vi "Set String Constant Value.vi"(8 "Error In":errorcluster, 9 "Value":string, 10 "Label":string, 11 "VI Path":path) -> (0 "Error Out":errorcluster)   [LabVIEW 2011, in "Generator.lvlib"]
doc: "This VI sets the value of a labeled string constant."
uses:
  Generator.lvlib
  <vilib>/Utility/traverseref.llb/TRef TravTarget.ctl
  <vilib>/Utility/traverseref.llb/VI Scripting - Traverse.lvlib
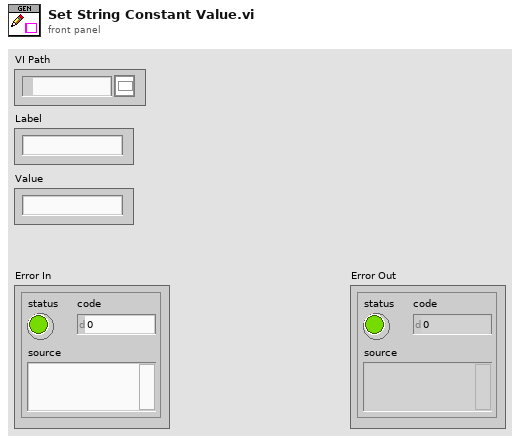
[diagram p1: front panel]
types:
  T1 = typedef "TRef TravTarget.ctl" = enum16{"FP", "BD", "Other"}
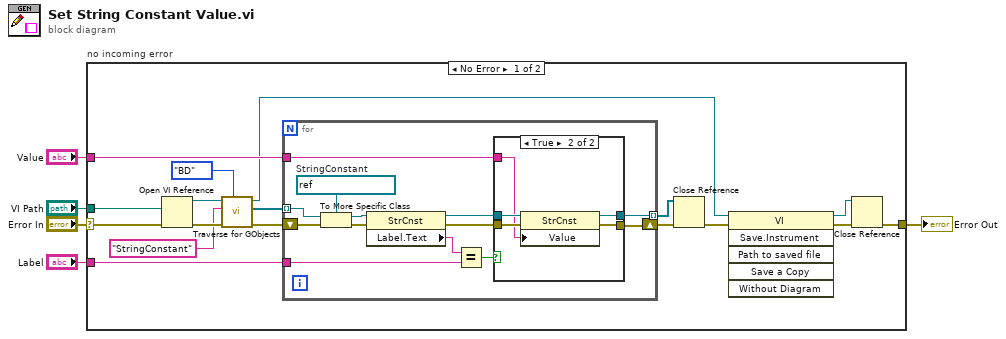
[diagram p0: block diagram]
diagram:
  n1 = case "no incoming error" shown="No Error" "Error In" {
    selector: "Error In" -> [w22 w43]
    tunnel: [w6 w43] -> w4
    tunnel: "VI Path" -> [w21 _]
    tunnel: "Label" -> [w14 _]
    tunnel: "Value" -> [w13 _]
    frame No Error {
      n2 = Open VI Reference(vi path=w21, error in (no error)=w22) -> (vi reference=w19:refnum<vi>, error out=w20:errorcluster)  [unwired: 4 in]
      n3 = call <vilib>:"Traverse for GObjects.vi"("Traverse Target"=TRef_TravTarget."BD", "error in (no error)"=w20, "Class Name"="StringConstant", "VI Refnum"=w19) -> ("error out"=w16:errorcluster, "References"=w15:refnum<vi>[], "dup VI Refnum"=w9:refnum<vi>)  [unwired: 4 in, 1 out]
      n4 = for {
        shift-right: [w23] -> w12
        shift-left: w16 -> [w35]
        tunnel: w15 -> [w34] mode=indexing
        tunnel: w14 -> [w29]
        tunnel: w13 -> [w25]
        tunnel: [w24] -> w11 mode=indexing
        w33 = refnum<vi> refnum  # StringConstant
        n5 = To More Specific Class(target class=w33, reference=w34, error in=w35) -> (specific class reference=w31:refnum<vi>, error out=w32:errorcluster)
        n6 = property class="StrCnst"(reference=w31, error in=w32) -> (reference out=w26:refnum<vi>, error out=w28:errorcluster, "Label.Text"=w30:string)
        n7 = Equal?(x=w30, y=w29) -> (x = y?=w27:bool)
        n8 = case shown="True" w27 {
          tunnel: w28 -> [w36 w41]
          tunnel: w26 -> [w37 w42]
          tunnel: w25 -> [_ w40]
          tunnel: [w36 w39] -> w23
          tunnel: [w37 w38] -> w24
          frame False {
          }
          frame True {
            n9 = property class="StrCnst"(reference=w42, error in=w41, "Value"=w40) -> (reference out=w38:refnum<vi>, error out=w39:errorcluster)
          }
        }
      }
      n10 = Close Reference(reference=w11, error in (no error)=w12) -> (error out=w10:errorcluster)
      n11 = invoke class="VI" method="Save.Instrument"(reference=w9, error in=w10) -> (reference out=w7:refnum<vi>, error out=w8:errorcluster)  [unwired: 4 in, 4 out]
      n12 = Close Reference(reference=w7, error in (no error)=w8) -> (error out=w6:errorcluster)
    }
    frame Error {
    }
  }
  "Error Out" <- w4
